vi "数组案例之数字个数计算(下).vi"() -> ()   [LabVIEW 2018]
panel:
  out "转置的数组":dbl[][](array[numeric])
  out "数组 3":dbl[](array[numeric])
  out "数组 2":dbl[](array[numeric])
  out "已排序的数组":dbl[](array[numeric])
  in  "数组":dbl[](array[numeric])
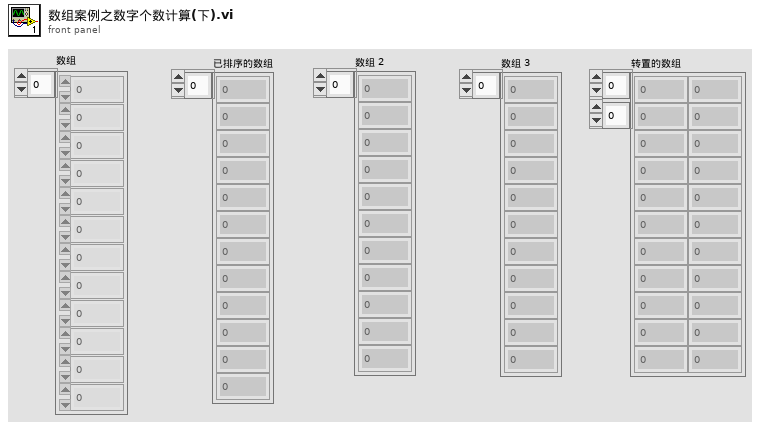
[diagram p1: front panel]
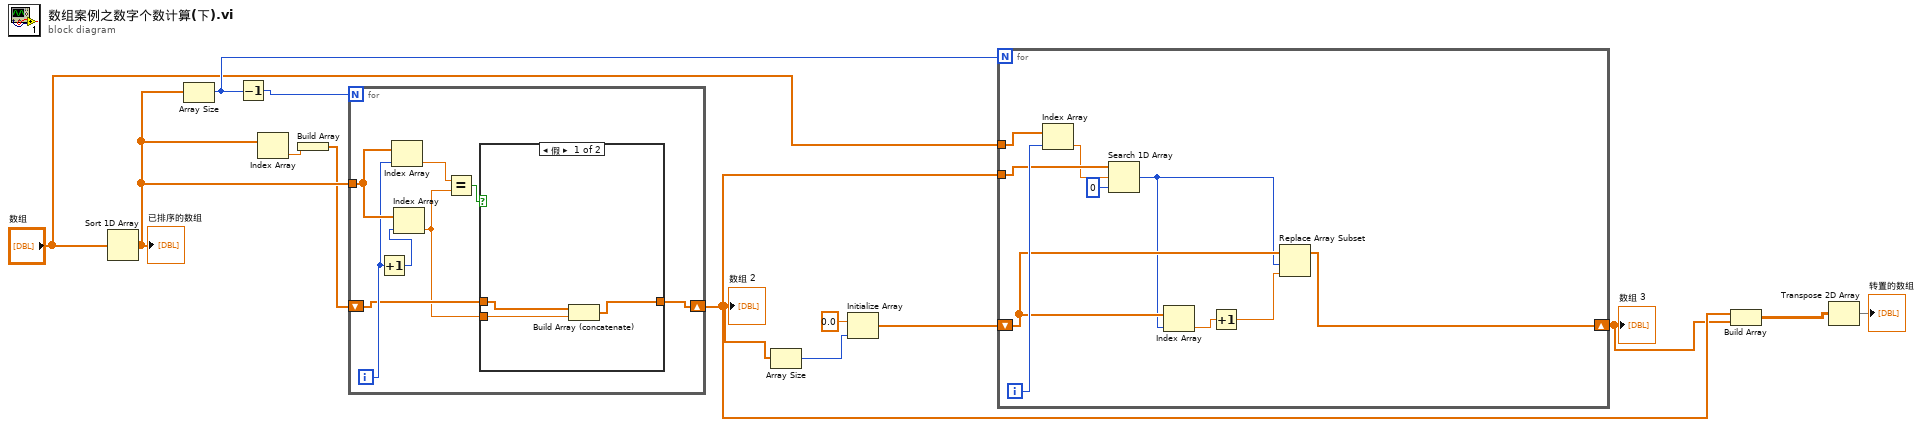
[diagram p0: block diagram]
diagram:
  n1 = Sort 1D Array(array="数组") -> (sorted array=w12:dbl[])
  "已排序的数组" <- w12
  n2 = Array Size(array=w12) -> (size(s)=w9:i32)
  n3 = Decrement(x=w9) -> (x-1=w13:i32)
  n4 = Index Array(array=w12) -> (element=w11:dbl)  [unwired: 1 in]
  n5 = Build Array(w11) -> (w10:dbl[])
  n6 = for {
    N: w13 -> [_]
    tunnel: w12 -> [w21]
    shift-right: [w15] -> w4
    shift-left: w10 -> [w16]
    i -> [w19]
    n7 = Increment(x=w19) -> (x+1=w20:i32)
    n8 = Index Array(array=w21, index=w19) -> (element=w18:dbl)
    n9 = Index Array(array=w21, index=w20) -> (element=w14:dbl)
    n10 = Equal?(x=w18, y=w14) -> (x = y?=w17:bool)
    n11 = case shown="假" w17 {
      tunnel: w16 -> [w24 w25]
      tunnel: [w22 w25] -> w15
      tunnel: w14 -> [w23 _]
      frame False {
        n12 = Build Array (concatenate)(w24, w23) -> (w22:dbl[])
      }
      frame True {
      }
    }
  }
  "数组 2" <- w4
  n13 = Array Size(array=w4) -> (size(s)=w6:i32)
  n14 = Initialize Array(0.0 ("元素"), w6) -> (w5:dbl[])
  n15 = for {
    N: w9 -> [_]
    tunnel: "数组" -> [w35]
    tunnel: w4 -> [w33]
    shift-right: [w26] -> w3
    shift-left: w5 -> [w29]
    i -> [w34]
    n16 = Index Array(array=w35, index=w34) -> (element=w32:dbl)
    n17 = Search 1D Array(1D array=w33, element=w32, start index (0)=0 ("开始索引(0)")) -> (index of element=w28:i32)
    n18 = Index Array(array=w29, index=w28) -> (element=w30:dbl)
    n19 = Increment(x=w30) -> (x+1=w27:dbl)
    n20 = Replace Array Subset(array=w29, new element=w27, index=w28) -> (w26:dbl[])
  }
  "数组 3" <- w3
  n21 = Build Array(w4, w3) -> (w2:dbl[][])
  n22 = Transpose 2D Array(2D array=w2) -> (transposed array=→"转置的数组":dbl[][])
